vi "vSwap_e.vi"(2 "v Ctrl in":refnum<class "CtrlLine.lvclass">[](array[class]), 7 "QuWire in":refnum<class "QuWire.lvclass">) -> (8 "QuWire out":refnum<class "QuWire.lvclass">, 13 "v Swap out":refnum<class "CtrlLine.lvclass">)   [LabVIEW 2020]
doc: "SWAP Gate (should be paired with an other qubit)\n\nExchanges the states of two qubits. \n\nMatrix: [[ 1, 0, 0, 0], [ 0, 0, 1, 0], [ 0, 1, 0, 0], [ 0, 0, 0, 1]]"
uses:
  QuSim/QuWire/QuWire.lvclass
  QuSim/QuWire/CtrlLine/CtrlLine.lvclass
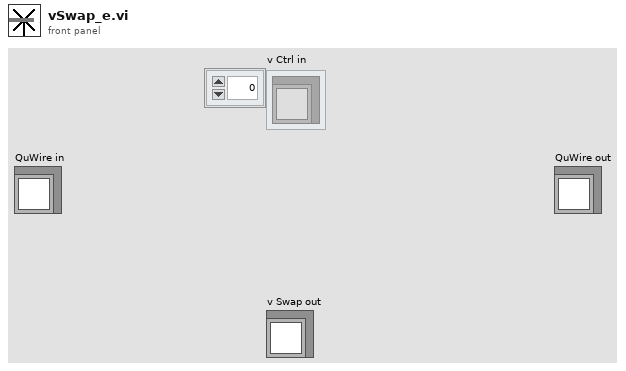
[diagram p1: front panel]
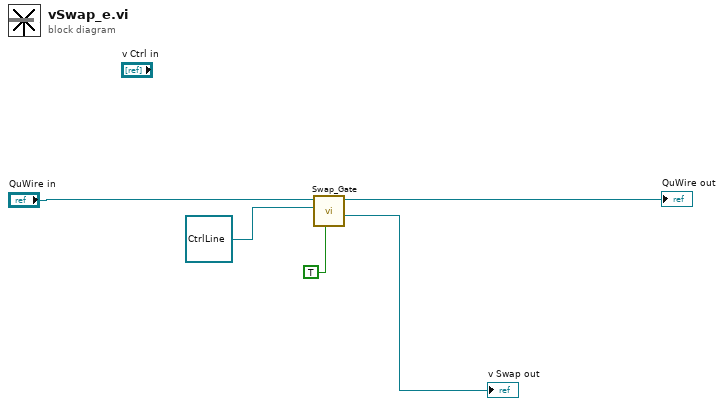
[diagram p0: block diagram]
diagram:
  n1 = call "Swap_Gate.vi"("Top Gate?"=TRUE, "u CtrlLine in"=refnum<class "CtrlLine.lvclass"> refnum ("u Ctrl Line in"), "QuWire in"="QuWire in") -> ("d CtrlLine out"=→"v Swap out":refnum<class "CtrlLine.lvclass">, "QuWire out"=→"QuWire out":refnum<class "QuWire.lvclass">)  [unwired: 6 in, 1 out]
